vi "OriginalDigitizerLive.vi"() -> ()   [LabVIEW 2020]
doc: "Example Description:\nThis example demonstrates how to enable Time Interleaved Sampling with the NI 5772 adapter module to achieve a sampling rate of 1.6GS/s. This example continuously acquires records of analog input data from the NI 5772 adapter module. It allows you to select an AI channel, trigger type, and record size. This VI must be compiled before it is run. \n\nRunning the VI:\nThis VI must be run from the NI 5772 - Getting Started (Host).vi. Refer to the host VI documentation for steps regarding running and configuring the FPGA VI. \n\nExecution Steps:\nRefer to the Block Diagram of this VI for execution comments."
uses:
  Controls/AI Trigger Type.ctl
  Controls/Aquire State.ctl
  Controls/NeighbouringAvgStates.ctl
  <vilib>/Platform/TimedLoop/XDataNode/timing_clust.ctl
  <vilib>/Platform/TimedLoop/XDataNode/nitl_modes.ctl
  <vilib>/Platform/TimedLoop/XDataNode/wakeup.ctl
  <vilib>/rvi/Emulation/niFpgaGetClockAttributes.vi
  <vilib>/rvi/Emulation/niFpgaSctlEmulationGetInTimedLoop.vi
  <vilib>/rvi/Emulation/niFpgaEmulationReportErrorSimple.vi
  <vilib>/rvi/eio/common/nirviEmuTemplateMethod_errors.vi
  <vilib>/rvi/Emulation/niFpgaCriticalErrorInLSC.vi
  <vilib>/rvi/interface/RandomDataEmulation/niFpgaRandomDataHandleErrors.vi
  <vilib>/rvi/Emulation/niFpgaEmulationIsFPGAContextNoSignature.vi
  <vilib>/rvi/errors/niFpgaSetErrorForExecOnDevCompSimple.vi
  <vilib>/rvi/eio/common/nirviEmuReportErrorAndStop.vi
  <vilib>/rvi/DataTransferAndStorage/Container/Common/niFpgaContainerGetUniqueNameForEmu.vi
  <vilib>/rvi/FIFO/Fifo_Resource/nirvififoEmulationSetSize.vi
  <vilib>/rvi/FIFO/Fifo_Resource/nirviFifoEmulationQueueMgr.vi
  <instcachedir>/0/nirviFifoEmulationQueueMgr_E5CAEC123FF24DC58D834DCA3CDAA9B5.lvgen/nirviFifoEmulationQueueMgr_E5CAEC123FF24DC58D834DCA3CDAA9B5_000.vi
  <vilib>/Utility/error.llb/Clear Errors.vi
  <vilib>/rvi/FIFO/Fifo_Resource/nirvififoEmulationCreateLock.vi
  <vilib>/rvi/Emulation/niFpgaProcessEmulError.vi
  <vilib>/rvi/FIFO/Fifo_Resource/nirvififoEmulationObtainLock.vi
  <vilib>/rvi/FIFO/Fifo_Resource/nirvififoEmulationReleaseLock.vi
  <vilib>/rvi/occurrence/nirviWaitOnOccurrenceBase.vi
  <vilib>/rvi/errors/nirviReportUnexpectedCaseInternalError.vi
  <vilib>/rvi/errors/nirviReportUnexpectedCaseInternalError (U32).vi
  <vilib>/rvi/FIFO/Fifo_Resource/nirvififoEmulationDetermineInputValidOut.vi
  <vilib>/eio/EIONode/EIONode.xnode
  <vilib>/Platform/TimedLoop/XDataNode/XDataNode.xnode
  <vilib>/rvi/DataTransferAndStorage/Container/XNode/niFpgaContainer.xnode
  <vilib>/rvi/interface/RandomDataEmulation/nirviRandomDataFpgaReadWriteTemplate.vi
  <vilib>/rvi/FIFO/Fifo_Resource/nirvififoEmulationRead.vi
  <vilib>/rvi/FIFO/Fifo_Resource/nirvififoEmulationWrite.vi
  <vilib>/Platform/TimedLoop/XDataNode/XDNodeRunTimeDep.lvlib
  <instrlib>/_niInstr/Basic Elements/v1/FPGA/niInstr Basic Elements v1 FPGA.lvlib
panel:
  in  "DS":u8
  in  "Trigger":bool=TRUE
  out "Acquire State":T1
  in  "Delay Cycles":u16=512 caption="Samples Per Trigger" min=1 step=1
  out "TS FIFO In Overflow?":bool caption="FIFO Overflow?"
  in  "Samples Per Trigger":u16=512 min=1 step=1
  in  "Arm Trigger":bool
  in  "User Command Commit":bool
  in  "User Command":u8
  out "User Command Idle":bool
  out "User Command Status":u8
  in  "User Data 0":u16
  in  "User Data 1":u8
  out "PLL Locked":bool
  out "User Error":bool
  out "Configured?":bool
  out "DMA FIFO Overflow?":bool caption="FIFO Overflow?"
  in  "Trigger Level":i16
  in  "Trigger Type":T2
  # "Resource Configuration"
  # "Refer to the Block Diagram of this VI for execution comments."
  # "For other instructions, select Help>>Show Context Help and move the cursor over the VI icon to display help for this VI."
  # "Analog Input"
  # "Clock Configuration"
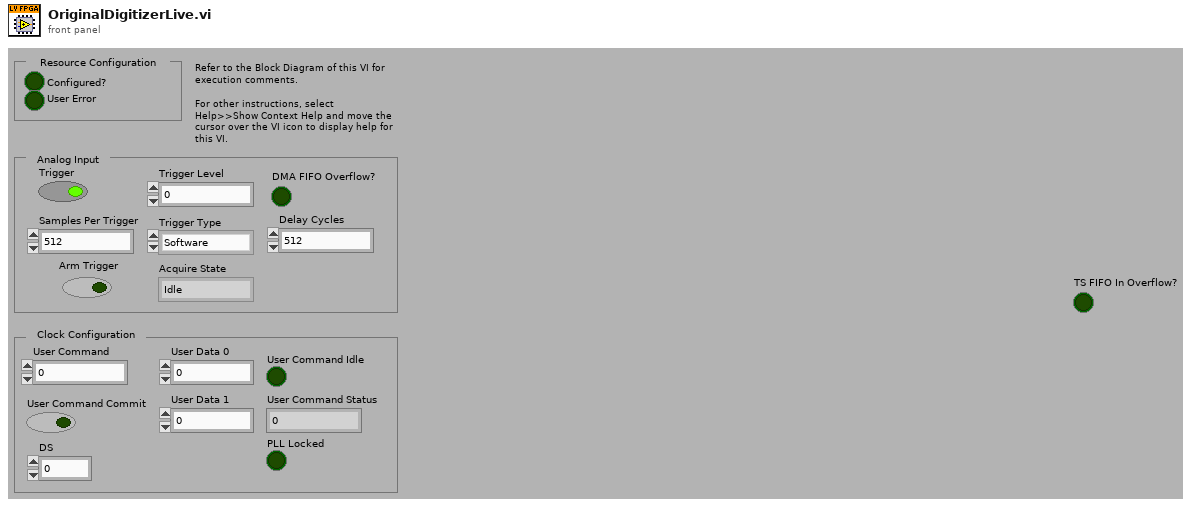
[diagram p1: front panel]
types:
  T1 = typedef "Aquire State.ctl" = enum8{"Idle", "Wait for Trigger", "AlignWave", "Hold Aquire", "Acquire", "WaitForWaveCompletion", "CheckAvg"}
  T2 = typedef "AI Trigger Type.ctl" = enum8{"Software", "Data Edge"}
  T3 = typedef "NeighbouringAvgStates.ctl" = enum16{"Read_noDS", "Write1_noDS", "Write2_noDS"}
  T4 = typedef "XDNodeRunTimeDep.lvlib/timing_clust.ctl" = cluster{"Expected End [f-1]":u64, "Actual End [f-1]":u64, "Finished Late? [f-1]":bool, "Expected End [i-1]":u64, "Actual End [i-1]":u64, "Finished Late? [i-1]":bool, "Expected Start [i]":u64, "Actual Start [i]":u64, "Expected Start [f]":u64, "Actual Start [f]":u64, "Source Name":string, "Structure Name":string, "Period":i64, "Deadline":i64, "Offset":i64, "Start":i64, "Priority":i32, "Timeout":i32, "Mode":T5, "Wakeup Reason":T6, "Error":errorcluster, "Source Type":string, "Secondary Source Type":string, "Global End Time":u64, "Global Start Time":u64, "Frame Duration":u64, "Iteration Duration":u64, "Assigned CPU":i32, "I/O Scan Engine Mode":u32}
  T5 = typedef "XDNodeRunTimeDep.lvlib/nitl_modes.ctl" = enum32{"No Change", "Process missed periods, maintain original phase", "Discard missed periods, maintain original phase", "Process missed periods, ignore original phase", "Discard missed periods, ignore original phase"}
  T6 = typedef "XDNodeRunTimeDep.lvlib/wakeup.ctl" = enum32{"Normal", "Aborted", "Asynchronous wakeup", "Timing source error", "Timed loop error", "Timeout"}
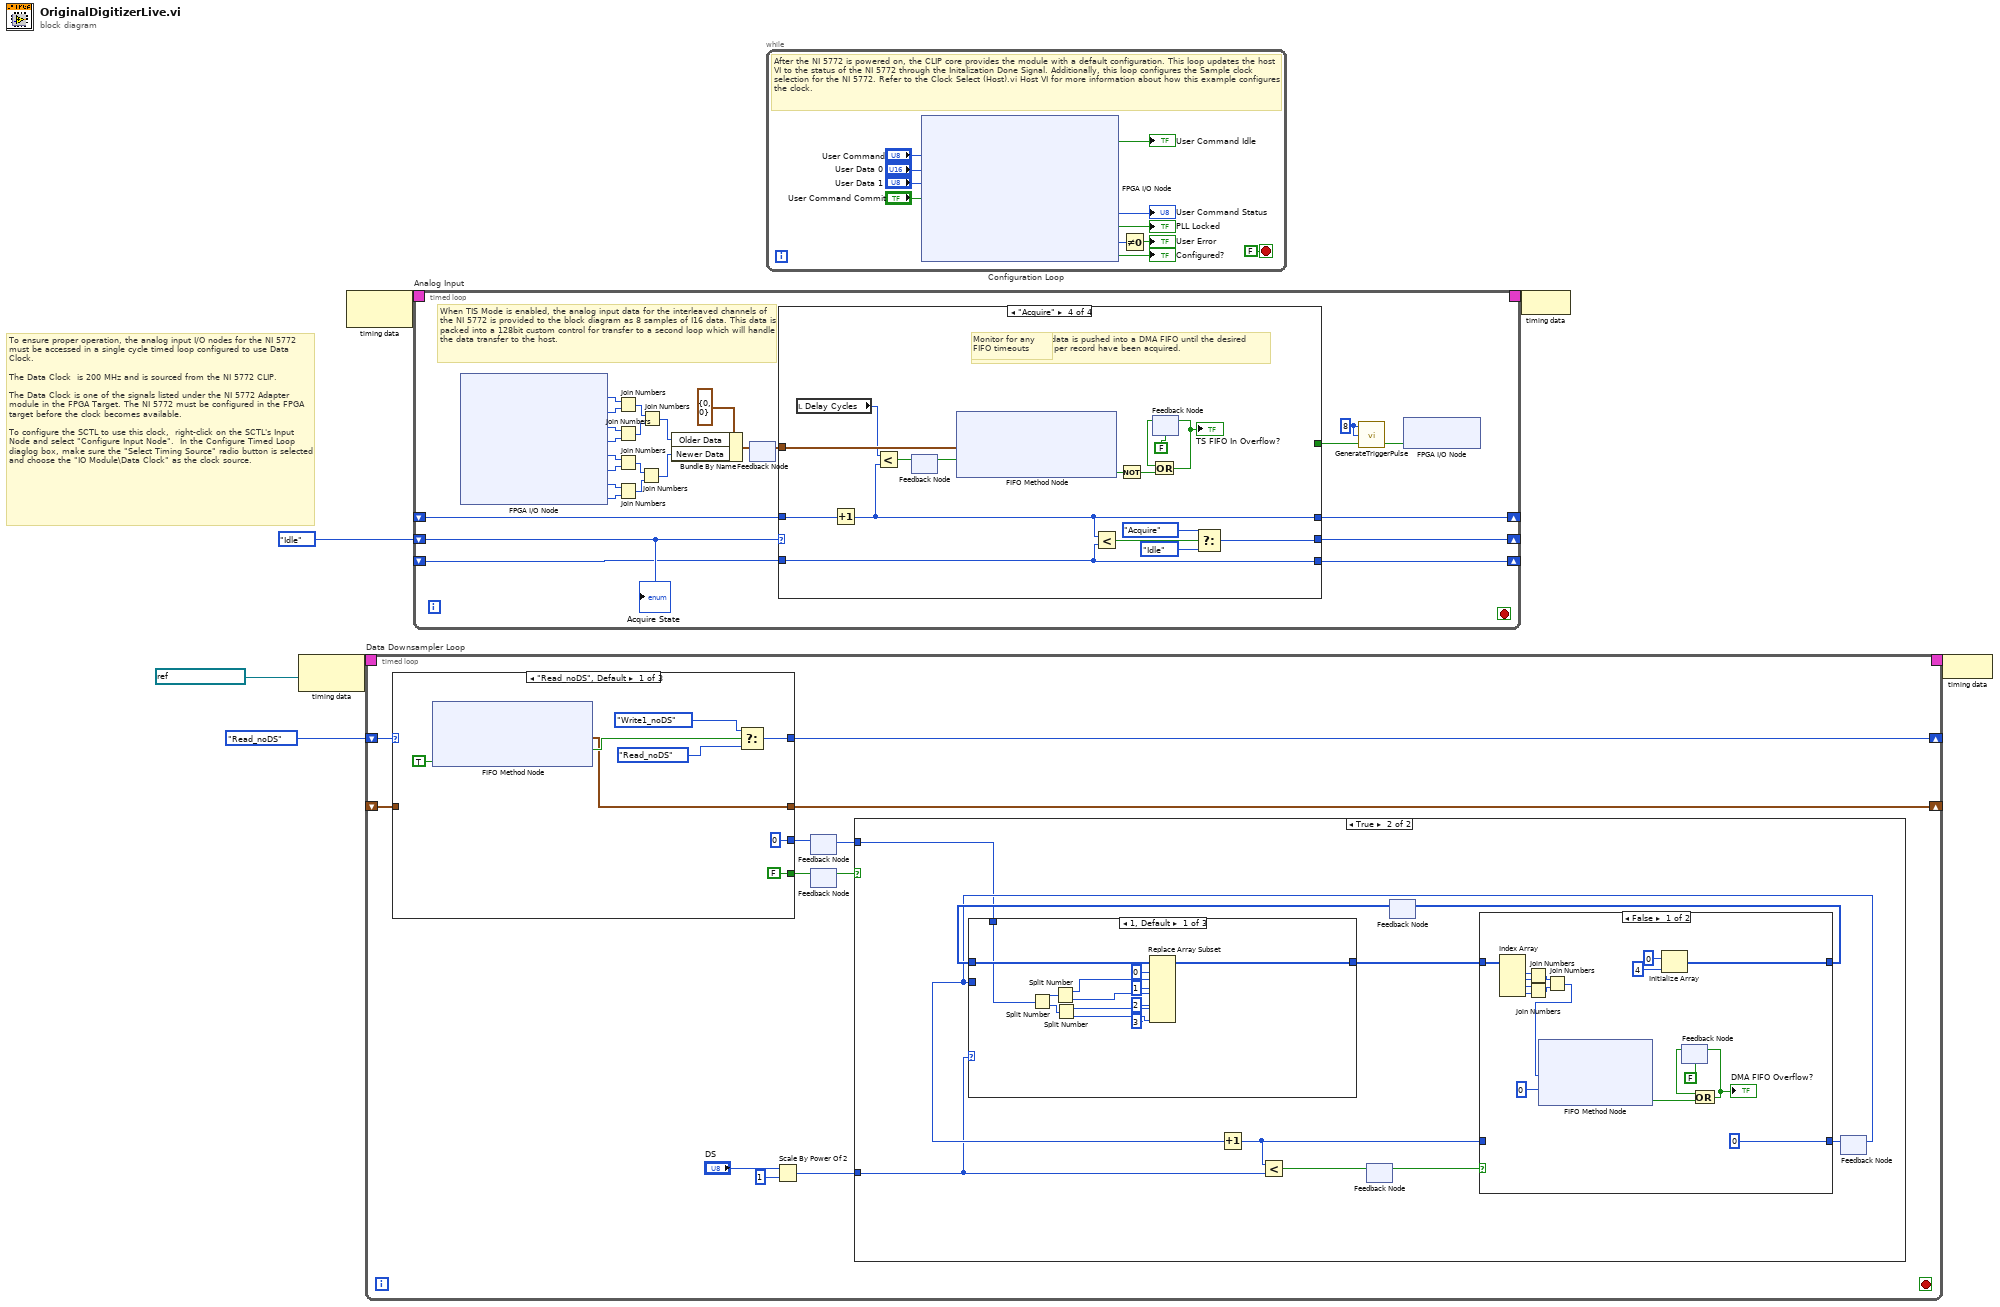
[diagram p0: block diagram]
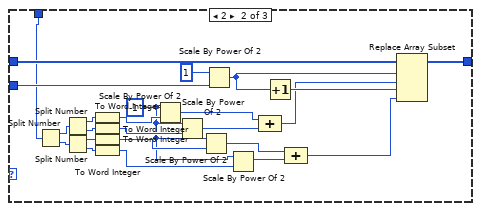
[diagram p4: hidden frame]
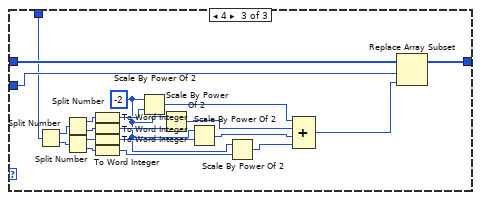
[diagram p5: hidden frame]
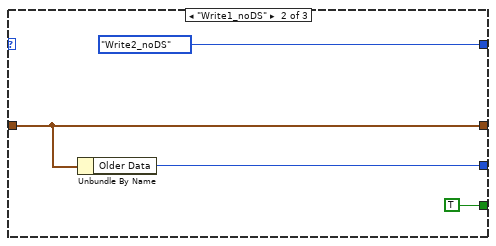
[diagram p6: hidden frame]
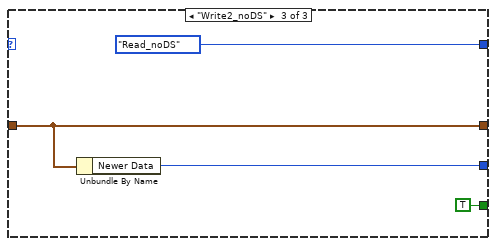
[diagram p7: hidden frame]
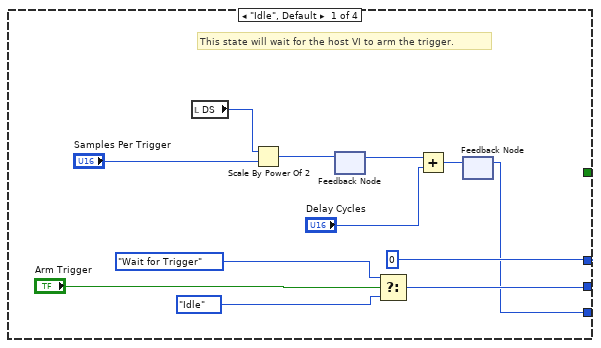
[diagram p8: hidden frame]
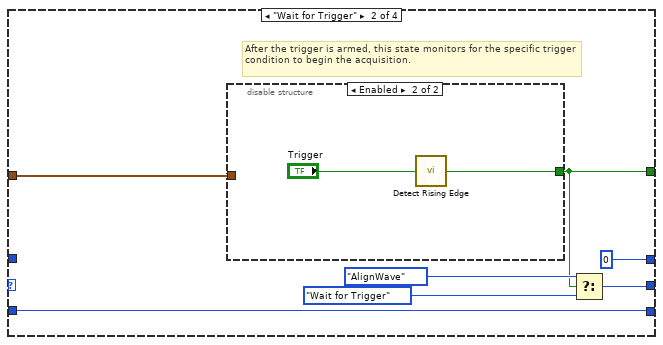
[diagram p9: hidden frame]
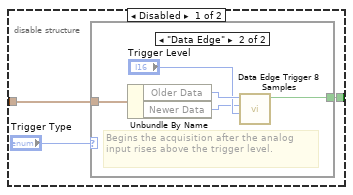
[diagram p10: hidden frame]
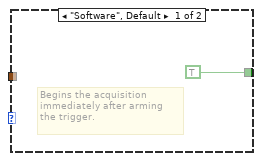
[diagram p11: hidden frame]
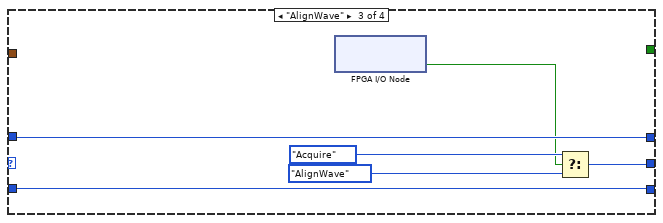
[diagram p12: hidden frame]
diagram:
  # "To ensure proper operation, the analog input I/O nodes for the NI 5772 must be accessed in a single cycle timed loop configured to use Data Clock. \n\nThe Data Clock  is 200 MHz and is sourced from the NI 5772 CLIP.\n\nThe Data Clock is one of the signals listed under the NI 5772 Adapter module in the FPGA Target. The NI 5772 must be configured in the FPGA target before the clock becomes available. \n\nTo configure the SCTL to use this clock,  right-click on the SCTL's Input Node and select \"Configure Input Node\".  In the Configure Timed Loop diaglog box, make sure the \"Select Timing Source\" radio button is selected and choose the \"IO Module\\Data Clock\" as the clock source."
  n1 = node-c288(refnum<k21> "200 MHz Clock" ("Source Name")) -> (w3:T4)
  n2 = node-c288() -> (w7:T4)  [unwired: 1 in]
  n3 = timed-loop "Data Downsampler Loop" {
    shift-right: [w17] -> _
    shift-left: NeighbouringAvgStates."Read_noDS" -> [w18]
    timing: w3 -> [_]
    timing-out: [_] -> w2
    shift-right: [w16] -> _
    shift-left: _ -> [w15]
    stop <- _ stop-if-true
    n4 = case shown="\"Read_noDS\", Default" w18 {
      tunnel: [w111 NeighbouringAvgStates."Write2_noDS" ("f") NeighbouringAvgStates."Read_noDS" ("f")] -> w17
      tunnel: [w107 w115 w119] -> w16
      tunnel: w15 -> [_ w115 w119]
      tunnel: [u64 0 ("Newer Data") w114 w118] -> w13
      tunnel: [FALSE ("Input Valid") TRUE ("Input Valid") TRUE ("Input Valid")] -> w14
      frame "Read_noDS", Default {
        n5 = xnode ("FIFO Method Node")("Ready for Output"=TRUE) -> ("Element"=w107:cluster{"Older Data":u64, "Newer Data":u64}, "Output Valid"=w110:bool)  [unwired: 1 in, 1 out]
        n6 = Select(t=NeighbouringAvgStates."Write1_noDS", s=w110, f=NeighbouringAvgStates."Read_noDS") -> (s? t:f=w111:T3)
      }
      frame "Write1_noDS" {
        n7 = Unbundle By Name(w115) -> ("Older Data"=w114:u64)
      }
      frame "Write2_noDS" {
        n8 = Unbundle By Name(w119) -> ("Newer Data"=w118:u64)
      }
    }
    n9 = Scale By Power Of 2(n="DS", x=u8 1) -> (x*2^n=w9:u8)
    n10 = feedback-in #1(w13) -> ()
    n11 = feedback #1() -> (w12:u64)  [unwired: 1 in]
    n12 = feedback-in #2(w14) -> ()
    n13 = feedback #2() -> (w11:bool)  [unwired: 1 in]
    n14 = case shown="True" w11 {
      tunnel: w12 -> [_ w21]
      tunnel: w9 -> [_ w19]
      frame False {
      }
      frame True {
        n15 = feedback #3() -> (w20:bool)  [unwired: 1 in]
        n16 = feedback #4() -> (w25:i16[])  [unwired: 1 in]
        n17 = feedback #5() -> (w22:u16)  [unwired: 1 in]
        n18 = case shown="1, Default" w19 {
          tunnel: w25 -> [w60 w78 w98]
          tunnel: [w59 w77 w97] -> w27
          tunnel: w22 -> [_ w74 w95]
          tunnel: w21 -> [w48 w61 w85]
          frame 1, Default {
            n19 = Split Number(x=w48) -> (hi(x)=w58:u32, lo(x)=w57:u32)
            n20 = Split Number(x=w58) -> (hi(x)=w56:u16, lo(x)=w55:u16)
            n21 = Split Number(x=w57) -> (hi(x)=w54:u16, lo(x)=w53:u16)
            n22 = Replace Array Subset(array=w60, new element #1=w56, index #1=0 ("index"), new element #2=w55, index #2=1 ("index"), new element #3=w54, index #3=2 ("index"), new element #4=w53, index #4=3 ("index")) -> (w59:i16[])
          }
          frame 2 {
            w66 = i16 -1 ("n")
            n23 = Split Number(x=w61) -> (hi(x)=w84:u32, lo(x)=w83:u32)
            n24 = Split Number(x=w84) -> (hi(x)=w82:u16, lo(x)=w81:u16)
            n25 = Split Number(x=w83) -> (hi(x)=w80:u16, lo(x)=w79:u16)
            n26 = To Word Integer(number=w82) -> (16bit integer=w70:i16)
            n27 = To Word Integer(number=w81) -> (16bit integer=w69:i16)
            n28 = To Word Integer(number=w80) -> (16bit integer=w68:i16)
            n29 = To Word Integer(number=w79) -> (16bit integer=w67:i16)
            n30 = Scale By Power Of 2(n=w66, x=w70) -> (x*2^n=w65:i16)
            n31 = Scale By Power Of 2(n=w66, x=w69) -> (x*2^n=w64:i16)
            n32 = Scale By Power Of 2(n=w66, x=w68) -> (x*2^n=w63:i16)
            n33 = Scale By Power Of 2(n=i16 1, x=w74) -> (x*2^n=w75:u16)
            n34 = Scale By Power Of 2(n=w66, x=w67) -> (x*2^n=w62:i16)
            n35 = Compound Arithmetic op=ADD(w65, w64) -> (w72:i16)
            n36 = Increment(x=w75) -> (x+1=w76:u16)
            n37 = Compound Arithmetic op=ADD(w63, w62) -> (w71:i16)
            n38 = Replace Array Subset(array=w78, new element #1=w72, index #1=w75, new element #2=w71, index #2=w76) -> (w77:i16[])
          }
          frame 4 {
            w86 = i16 -2 ("n")
            n39 = Split Number(x=w85) -> (hi(x)=w104:u32, lo(x)=w103:u32)
            n40 = Split Number(x=w104) -> (hi(x)=w102:u16, lo(x)=w101:u16)
            n41 = Split Number(x=w103) -> (hi(x)=w100:u16, lo(x)=w99:u16)
            n42 = To Word Integer(number=w102) -> (16bit integer=w93:i16)
            n43 = To Word Integer(number=w101) -> (16bit integer=w92:i16)
            n44 = To Word Integer(number=w100) -> (16bit integer=w91:i16)
            n45 = To Word Integer(number=w99) -> (16bit integer=w90:i16)
            n46 = Scale By Power Of 2(n=w86, x=w93) -> (x*2^n=w94:i16)
            n47 = Scale By Power Of 2(n=w86, x=w92) -> (x*2^n=w87:i16)
            n48 = Scale By Power Of 2(n=w86, x=w91) -> (x*2^n=w88:i16)
            n49 = Scale By Power Of 2(n=w86, x=w90) -> (x*2^n=w89:i16)
            n50 = Compound Arithmetic op=ADD(w94, w87, w88, w89) -> (w96:i16)
            n51 = Replace Array Subset(array=w98, new element=w96, index=w95) -> (w97:i16[])
          }
        }
        n52 = Increment(x=w22) -> (x+1=w28:u16)
        n53 = Less?(x=w28, y=w19) -> (x < y?=w26:bool)
        n54 = feedback-in #3(w26) -> ()
        n55 = case shown="False" w20 {
          tunnel: w27 -> [w39 w47]
          tunnel: [w36 w47] -> w24
          tunnel: w28 -> [_ w46]
          tunnel: [u16 0 w46] -> w23
          frame False {
            n56 = Index Array(array=w39) -> (element #1=w43:i16, element #2=w42:i16, element #3=w41:i16, element #4=w40:i16)  [unwired: 4 in]
            n57 = Join Numbers(hi=w43, lo=w42) -> ((hi.lo)=w45:u32)
            n58 = Join Numbers(hi=w41, lo=w40) -> ((hi.lo)=w44:u32)
            n59 = Join Numbers(hi=w45, lo=w44) -> ((hi.lo)=w30:u64)
            n60 = xnode ("FIFO Method Node")("Element"=w30, "Timeout"=0) -> ("Timed Out?"=w31:bool)  [unwired: 1 in, 1 out]
            n61 = Initialize Array(i16 0 ("element"), 4 ("dimension size")) -> (w36:i16[])
            n62 = feedback #6(FALSE) -> (w32:bool)
            n63 = Compound Arithmetic op=OR(w32, w31) -> (w29:bool)
            "DMA FIFO Overflow?" <- w29
            n64 = feedback-in #6(w29) -> ()
          }
          frame True {
          }
        }
        n65 = feedback-in #4(w24) -> ()
        n66 = feedback-in #5(w23) -> ()
      }
    }
  }
  n67 = timed-loop "Analog Input" {
    timing: w7 -> [_]
    timing-out: [_] -> w6
    shift-right: [w147] -> _
    shift-left: Aquire_State."Idle" ("Acquire State") -> [w137]
    shift-right: [w148] -> _
    shift-left: _ -> [w138]
    shift-right: [w146] -> _
    shift-left: _ -> [w136]
    stop <- _ stop-if-true
    w124 = u16 8 ("Pulse Width On [cycles]")
    # "When TIS Mode is enabled, the analog input data for the interleaved channels of the NI 5772 is provided to the block diagram as 8 samples of I16 data. This data is packed into a 128bit custom control for transfer to a second loop which will handle the data transfer to the host."
    n68 = xnode "FPGA I/O Node"() -> ("IO Module\\AI 1 Data N-3"=w129:i16, "IO Module\\AI 0 Data N-3"=w128:i16, "IO Module\\AI 1 Data N-2"=w127:i16, "IO Module\\AI 0 Data N-2"=w126:i16, "IO Module\\AI 1 Data N-1"=w130:i16, "IO Module\\AI 0 Data N-1"=w131:i16, "IO Module\\AI 1 Data N"=w132:i16, "IO Module\\AI 0 Data N"=w133:i16)  [unwired: 8 in, 8 out]
    n69 = Join Numbers(hi=w129, lo=w128) -> ((hi.lo)=w141:u32)
    n70 = Join Numbers(hi=w127, lo=w126) -> ((hi.lo)=w143:u32)
    n71 = Join Numbers(hi=w130, lo=w131) -> ((hi.lo)=w142:u32)
    n72 = Join Numbers(hi=w132, lo=w133) -> ((hi.lo)=w144:u32)
    n73 = Join Numbers(hi=w142, lo=w144) -> ((hi.lo)=w134:u64)
    n74 = Join Numbers(hi=w141, lo=w143) -> ((hi.lo)=w135:u64)
    n75 = Bundle By Name(cluster=cluster{"Older Data":u64, "Newer Data":u64} {"Older Data"=0, "Newer Data"=0} ("Element"), "Older Data"=w135, "Newer Data"=w134) -> (w139:cluster{"Older Data":u64, "Newer Data":u64})
    n76 = feedback #7() -> (w145:cluster{"Older Data":u64, "Newer Data":u64})  [unwired: 1 in]
    n77 = feedback-in #7(w139) -> ()
    n78 = case shown="\"Acquire\"" w137 {
      tunnel: [u16 0 u16 0 w181 w192] -> w148
      tunnel: w138 -> [_ _ w181 w200]
      tunnel: [w157 w163 w182 w198] -> w147
      tunnel: [w154 w167 w180 w195] -> w146
      tunnel: w136 -> [_ w167 w180 w195]
      tunnel: w145 -> [_ w166 _ w194]
      tunnel: [_ w161 _ _] -> w123
      frame "Idle", Default {
        # "This state will wait for the host VI to arm the trigger."
        n79 = local read "DS"() -> (w150:u8)
        n80 = Scale By Power Of 2(n=w150, x="Samples Per Trigger") -> (x*2^n=w152:u16)
        n81 = feedback-in #8(w152) -> ()
        n82 = feedback #8() -> (w149:u16)  [unwired: 1 in]
        n83 = Select(t=Aquire_State."Wait for Trigger" ("Acquire State"), s="Arm Trigger", f=Aquire_State."Idle" ("Acquire State")) -> (s? t:f=w157:T1)
        n84 = Add(x=w149, y="Delay Cycles") -> (x+y=w155:u16)
        n85 = feedback-in #9(w155) -> ()
        n86 = feedback #9() -> (w154:u16)  [unwired: 1 in]
      }
      frame "Wait for Trigger" {
        # "After the trigger is armed, this state monitors for the specific trigger condition to begin the acquisition."
        n87 = disable-structure shown="Enabled" {
          disable-tunnel: w166 -> [w169 _]
          disable-tunnel: [w168 w177] -> w161
          frame Disabled {
            n88 = case shown="\"Data Edge\"" "Trigger Type" {
              tunnel: w169 -> [_ w176]
              tunnel: [TRUE ("Trigger") w175] -> w168
              frame "Software", Default {
                # "Begins the acquisition immediately after arming the trigger."
              }
              frame "Data Edge" {
                # "Begins the acquisition after the analog input rises above the trigger level."
                n89 = Unbundle By Name(w176) -> ("Older Data"=w174:u64, "Newer Data"=w172:u64)
                n90 = call "Data Edge Trigger 8 Samples.vi"("Trigger Level"="Trigger Level", "Newer Data In"=w172, "Older Data In"=w174) -> ("Trigger"=w175:bool)  [unwired: 8 in]
              }
            }
          }
          frame Enabled {
            n91 = call <instrlib>:"Detect Rising Edge.vi"("signal"="Trigger") -> ("edge detected"=w177:bool)  [unwired: 14 in]
          }
        }
        n92 = Select(t=Aquire_State."AlignWave" ("Acquire State"), s=w161, f=Aquire_State."Wait for Trigger") -> (s? t:f=w163:T1)
      }
      frame "AlignWave" {
        n93 = xnode "FPGA I/O Node"() -> ("PXI_Trig0"=w179:bool)  [unwired: 1 in, 1 out]
        n94 = Select(t=Aquire_State."Acquire" ("Acquire State"), s=w179, f=Aquire_State."AlignWave") -> (s? t:f=w182:T1)
      }
      frame "Acquire" {
        # "Monitor for any  FIFO timeouts"
        # "While in this state, data is pushed into a DMA FIFO until the desired number of samples per record have been acquired."
        n95 = local read "Delay Cycles"() -> (w193:u16)
        n96 = Increment(x=w200) -> (x+1=w192:u16)
        n97 = Less?(x=w193, y=w192) -> (x < y?=w188:bool)
        n98 = feedback-in #10(w188) -> ()
        n99 = feedback #10() -> (w185:bool)  [unwired: 1 in]
        n100 = xnode ("FIFO Method Node")("Element"=w194, "Input Valid"=w185) -> ("Ready for Input"=w187:bool)  [unwired: 1 in, 1 out]
        n101 = Less?(x=w192, y=w195) -> (x < y?=w199:bool)
        n102 = Not(x=w187) -> (.not. x?=w186:bool)
        n103 = feedback #11(FALSE) -> (w189:bool)
        n104 = Or(x=w189, y=w186) -> (x .or. y?=w190:bool)
        "TS FIFO In Overflow?" <- w190
        n105 = feedback-in #11(w190) -> ()
        n106 = Select(t=Aquire_State."Acquire" ("Acquire State"), s=w199, f=Aquire_State."Idle" ("Acquire State")) -> (s? t:f=w198:T1)
      }
    }
    n107 = call "GenerateTriggerPulse.vi"("Trigger"=w123, "Pulse Width Off [cycles]"=w124, "Pulse Width On [cycles]"=w124) -> ("Out"=w125:bool)  [unwired: 2 out]
    n108 = xnode "FPGA I/O Node"("PXI_Trig1"=w125) -> ()  [unwired: 1 in, 1 out]
    "Acquire State" <- w137
  }
  n109 = while "Configuration Loop" {
    stop <- FALSE stop-if-true
    # "After the NI 5772 is powered on, the CLIP core provides the module with a default configuration. This loop updates the host VI to the status of the NI 5772 through the Initalization Done Signal. Additionally, this loop configures the Sample clock selection for the NI 5772. Refer to the Clock Select (Host).vi Host VI for more information about how this example configures the clock."
    n110 = xnode "FPGA I/O Node"("IO Module\\User Command"="User Command", "IO Module\\User Data 0"="User Data 0", "IO Module\\User Data 1"="User Data 1", "IO Module\\User Command Commit"="User Command Commit") -> ("IO Module\\User Command Idle"=→"User Command Idle":bool, "IO Module\\User Command Status"=→"User Command Status":u8, "IO Module\\PLL Locked"=→"PLL Locked":bool, "IO Module\\User Error"=w208:u8, "IO Module\\Initialization Done"=→"Configured?":bool)  [unwired: 9 in, 9 out]
    n111 = Not Equal To 0?(x=w208) -> (x != 0?=→"User Error":bool)
  }
  n112 = node-c288(w6) -> ()
  n113 = node-c288(w2) -> ()
